vi "test_libssh2_session_disconnect.vi"() -> ()   [LabVIEW 2013, in "libssh2_integration_tests.lvlib"]
uses:
  libssh2_integration_tests.lvlib
  libssh2/libssh2_init_default.vi
  libssh2/libssh2_session_handshake_tcp.vi
  libssh2/libssh2.lvlib
  <vilib>/addons/_JKI Toolkits/Caraya/classes/Test/Test.lvclass
  support/support.lvlib
  <vilib>/addons/_JKI Toolkits/Caraya/classes/Assert/Assert.lvclass
panel:
  out "error out":errorcluster
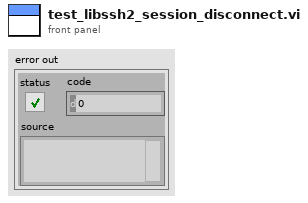
[diagram p1: front panel]
types:
  T1 = typedef "libssh2.lvlib/Session Refnum.ctl" = refnum<k1>
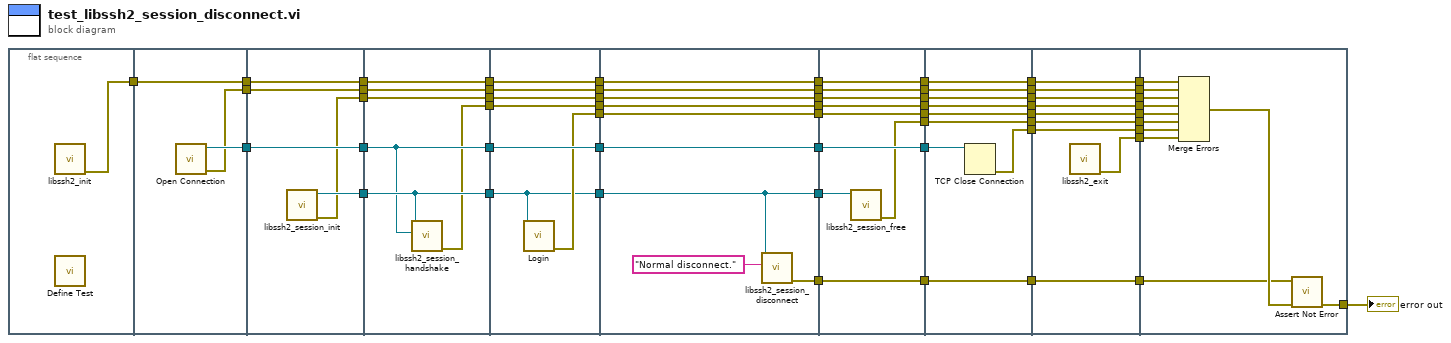
[diagram p0: block diagram]
diagram:
  n1 = flat-sequence {
    tunnel: [w57] -> w56
    tunnel: [w60] -> w55
    tunnel: w56 -> [w59]
    tunnel: [w59] -> w54
    tunnel: [w58] -> w53
    tunnel: w55 -> [w65]
    tunnel: [w65] -> w16
    tunnel: w54 -> [w64]
    tunnel: [w64] -> w15
    tunnel: w53 -> [w63]
    tunnel: [w63] -> w14
    tunnel: [w62] -> w13
    tunnel: [w61] -> w12
    tunnel: w16 -> [w67]
    tunnel: [w67] -> w41
    tunnel: w15 -> [w71]
    tunnel: [w71] -> w40
    tunnel: w14 -> [w70]
    tunnel: [w70] -> w39
    tunnel: [w69] -> w38
    tunnel: w13 -> [w69]
    tunnel: w12 -> [w68]
    tunnel: [w68] -> w37
    tunnel: [w66] -> w36
    tunnel: w41 -> [w78]
    tunnel: [w78] -> w24
    tunnel: w40 -> [w77]
    tunnel: [w77] -> w23
    tunnel: w39 -> [w76]
    tunnel: [w76] -> w22
    tunnel: w38 -> [w72]
    tunnel: w37 -> [w75]
    tunnel: [w75] -> w21
    tunnel: w36 -> [w74]
    tunnel: [w74] -> w20
    tunnel: [w73] -> w19
    tunnel: [w72] -> w18
    tunnel: w24 -> [w87]
    tunnel: [w87] -> w8
    tunnel: w23 -> [w86]
    tunnel: [w86] -> w7
    tunnel: w22 -> [w85]
    tunnel: [w85] -> w6
    tunnel: w21 -> [w84]
    tunnel: [w84] -> w5
    tunnel: w20 -> [w83]
    tunnel: [w83] -> w4
    tunnel: w19 -> [w82]
    tunnel: [w82] -> w3
    tunnel: w18 -> [w80]
    tunnel: [w81] -> w2
    tunnel: [w80] -> w1
    tunnel: w8 -> [w96]
    tunnel: [w96] -> w33
    tunnel: w7 -> [w95]
    tunnel: [w95] -> w32
    tunnel: w6 -> [w94]
    tunnel: [w94] -> w31
    tunnel: w5 -> [w93]
    tunnel: [w93] -> w30
    tunnel: w4 -> [w92]
    tunnel: [w92] -> w29
    tunnel: w3 -> [w91]
    tunnel: [w91] -> w28
    tunnel: [w90] -> w25
    tunnel: [w89] -> w9
    tunnel: w2 -> [w89]
    tunnel: w1 -> [w88]
    tunnel: w33 -> [w105]
    tunnel: w32 -> [w104]
    tunnel: [w104] -> w52
    tunnel: w31 -> [w103]
    tunnel: [w103] -> w51
    tunnel: [w102] -> w50
    tunnel: w30 -> [w101]
    tunnel: [w101] -> w49
    tunnel: w29 -> [w100]
    tunnel: [w100] -> w48
    tunnel: w28 -> [w99]
    tunnel: [w99] -> w35
    tunnel: [w98] -> w26
    tunnel: w25 -> [w98]
    tunnel: [w97] -> w10
    tunnel: w9 -> [w97]
    tunnel: w52 -> [w114]
    tunnel: [w114] -> w47
    tunnel: w51 -> [w113]
    tunnel: [w113] -> w46
    tunnel: w50 -> [w112]
    tunnel: [w112] -> w45
    tunnel: [w111] -> w44
    tunnel: w49 -> [w110]
    tunnel: [w110] -> w43
    tunnel: w48 -> [w109]
    tunnel: [w109] -> w42
    tunnel: w35 -> [w108]
    tunnel: [w108] -> w34
    tunnel: [w107] -> w27
    tunnel: w26 -> [w107]
    tunnel: [w106] -> w11
    tunnel: w10 -> [w106]
    tunnel: w47 -> [w125]
    tunnel: w46 -> [w124]
    tunnel: w45 -> [w123]
    tunnel: w44 -> [w122]
    tunnel: w43 -> [w121]
    tunnel: [w119] -> w17
    tunnel: w42 -> [w118]
    tunnel: w34 -> [w117]
    tunnel: w27 -> [w116]
    tunnel: w11 -> [w115]
    frame #0 {
      n2 = call-poly "libssh2_init.vi"() -> ("error out"=w57:errorcluster)  [unwired: 11 in]
      n3 = call <vilib>:"Define Test.vi"() -> ()  [unwired: 10 in, 2 out]
    }
    frame #1 {
      n4 = call "Open Connection.vi"() -> ("error out"=w58:errorcluster, "connection ID"=w60:refnum<k5>)  [unwired: 10 in]
    }
    frame #2 {
      n5 = call "libssh2_session_init.vi"() -> ("error out"=w61:errorcluster, "session"=w62:T1)  [unwired: 10 in]
    }
    frame #3 {
      n6 = call-poly "libssh2_session_handshake.vi"("tcp connection"=w67, "session"=w69) -> ("error out"=w66:errorcluster)  [unwired: 9 in]
    }
    frame #4 {
      n7 = call "Login.vi"("session"=w72) -> ("error out"=w73:errorcluster)  [unwired: 10 in]
    }
    frame #5 {
      n8 = call "libssh2_session_disconnect.vi"("description"="Normal disconnect.", "session"=w80) -> ("error out"=w81:errorcluster)  [unwired: 9 in]
    }
    frame #6 {
      n9 = call "libssh2_session_free.vi"("session"=w88) -> ("error out"=w90:errorcluster)  [unwired: 10 in]
    }
    frame #7 {
      n10 = TCP Close Connection(connection ID=w105) -> (error out=w102:errorcluster)  [unwired: 2 in, 1 out]
    }
    frame #8 {
      n11 = call "libssh2_exit.vi"() -> ("error out"=w111:errorcluster)  [unwired: 11 in]
    }
    frame #9 {
      n12 = Merge Errors(w125, w124, w121, w118, w117, w116, w123, w122) -> (w120:errorcluster)
      n13 = call <vilib>:"Assert Not Error.vi"("error in (no error)"=w120, "Not Error?"=w115) -> ("error out"=w119:errorcluster)  [unwired: 8 in, 1 out]
    }
  }
  "error out" <- w17
